vi "CS POLARIS BME DG Client.ProcCases.vi"(0 "i ref in":refnum<vi>, 1 "selector":string, 2 "Data":T1, 3 "call cluster":T2={"Object"="", "Selector"="", "CallType"=enum."synchronous", "Async Object"="", "Async Selector"="", "Data Descriptor"="", "Data"=[], "Error #"=0, "Expire"=0}, 5 "error in (no error)":errorcluster) -> (14 "i ref out":refnum<vi>, 17 "answer cluster":T2={"Object"="", "Selector"="", "CallType"=enum."synchronous", "Async Object"="", "Async Selector"="", "Data Descriptor"="", "Data"=[], "Error #"=0, "Expire"=0}, 19 "error out":errorcluster)   [LabVIEW 2009, in "CS POLARIS BME DG Client.lvlib"]
doc: "This method is called by a process from within the default case in the event loop. The methods of a class that are linked to events will be called from THIS method. Add your code here."
uses:
  CS POLARIS BME DG Client.lvlib
  CSCore/CSSystem/CoreDefs/CoreDefs.call_type.ctl
  CSCore/BaseProcess/BaseProcess.descriptor string definition.ctl
  CSCore/CSSystem/CoreDefs/CoreDefs.rawDataType.ctl
  CSCore/BaseProcess/BaseProcess.lvlib
  CSCore/CAEObj/CAEObj.lvlib
  lib.lib/UtilityLib/UtilityLib.lvlib
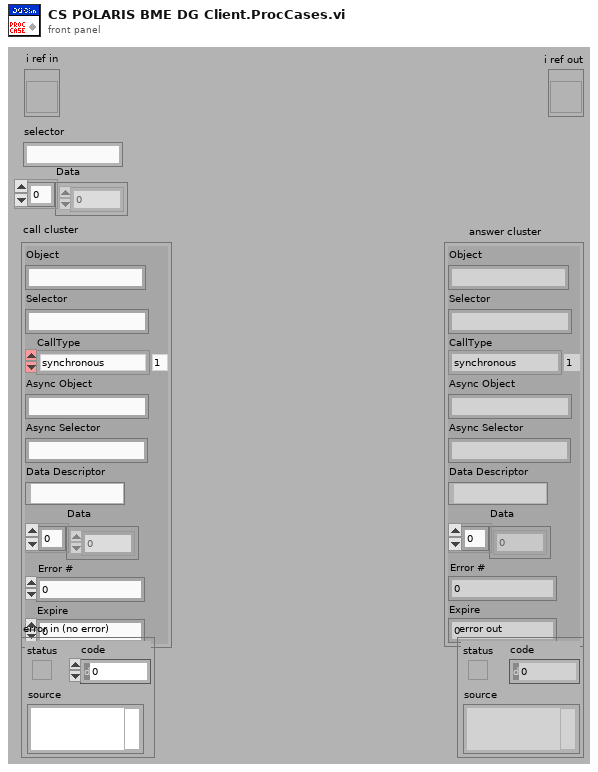
[diagram p1: front panel]
types:
  T1 = typedef "CoreDefs.rawDataType.ctl" = i8[]
  T2 = typedef "CoreDefs.call_type.ctl" = cluster{"Object":string, "Selector":string, "CallType":enum16{"simple", "synchronous", "asynchronous"}, "Async Object":string, "Async Selector":string, "Data Descriptor":T3, "Data":T1, "Error #":i32, "Expire":u32}
  T3 = typedef "BaseProcess.lvlib/BaseProcess.descriptor string definition.ctl" = string
  T4 = typedef "CS POLARIS BME DG Client.lvlib/CS POLARIS BME DG Client.i attribute.ctl" = cluster{"Delay Formula Ref":refnum<vi>, "Active Ref":refnum<vi>, "OutputModulo Ref":refnum<vi>, "Rep Rate Ref":refnum<vi>, "Next Shot Ref":refnum<vi>, "Error Ref":refnum<vi>, "Switch Ref":refnum<vi>, "New Delay Formula Ref":refnum<vi>, "New OutputModulo Ref ":refnum<vi>, "Channel":string, "CS DG Obj":string, "Stop Ref":refnum<vi>, "Max delay change":dbl, "Enabled fields":u8, "LockInfo Ref":refnum<vi>, "Next Common Shot Ref":refnum<vi>, "cur. abs del Ref":refnum<vi>, "new abs del Ref 2":refnum<vi>}
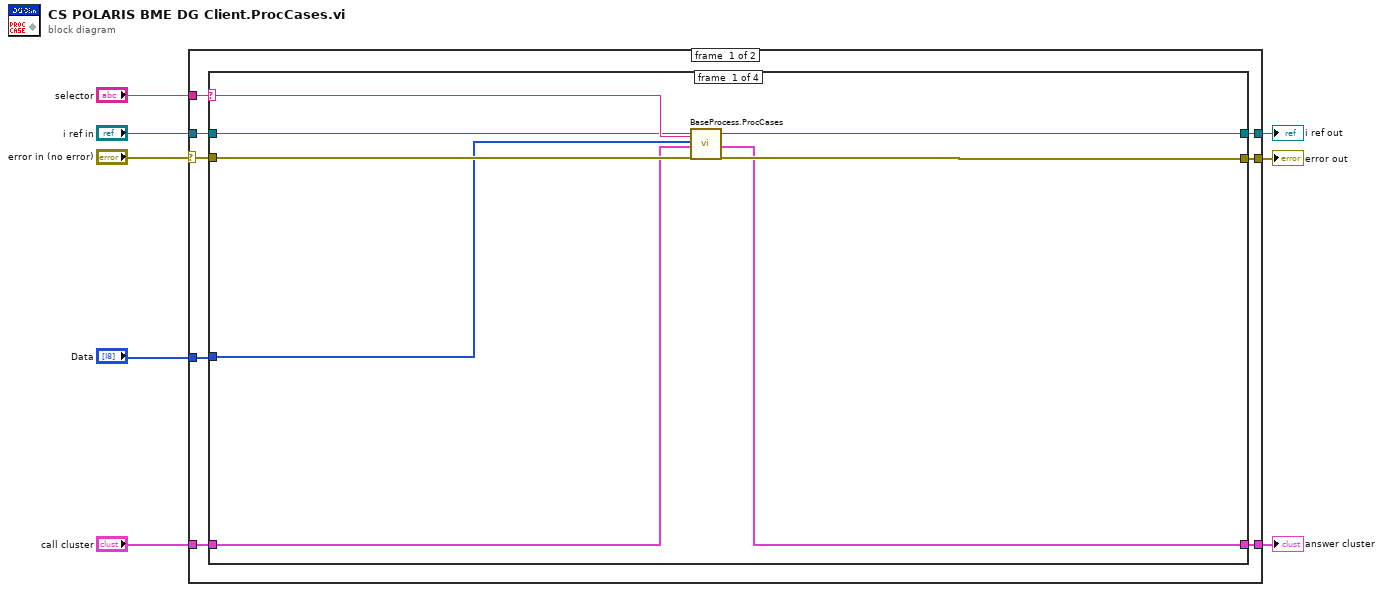
[diagram p0: block diagram]
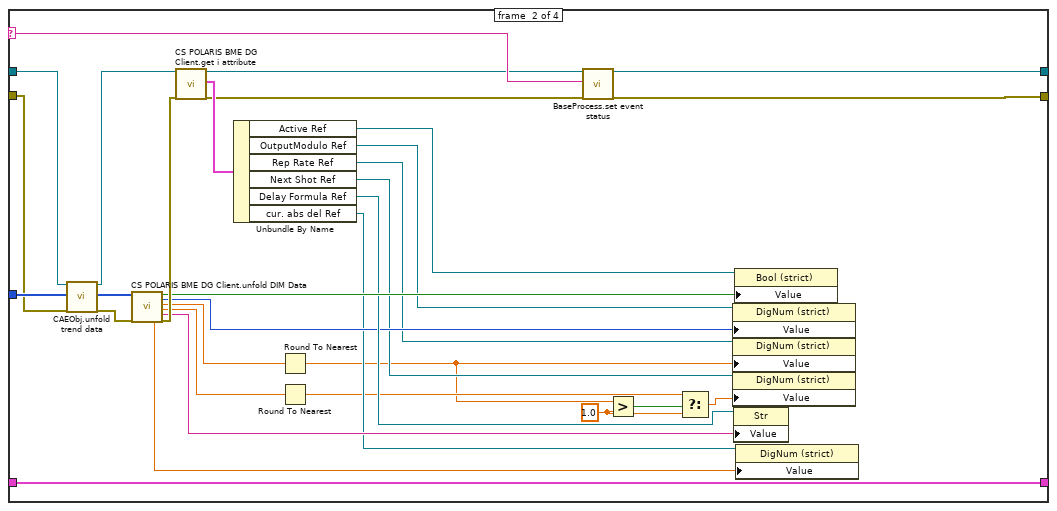
[diagram p2: hidden frame]
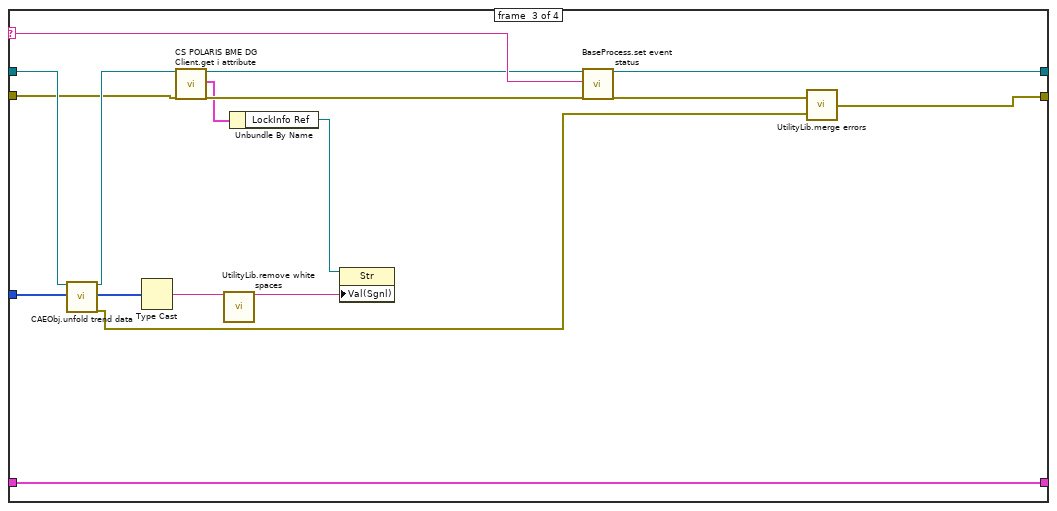
[diagram p3: hidden frame]
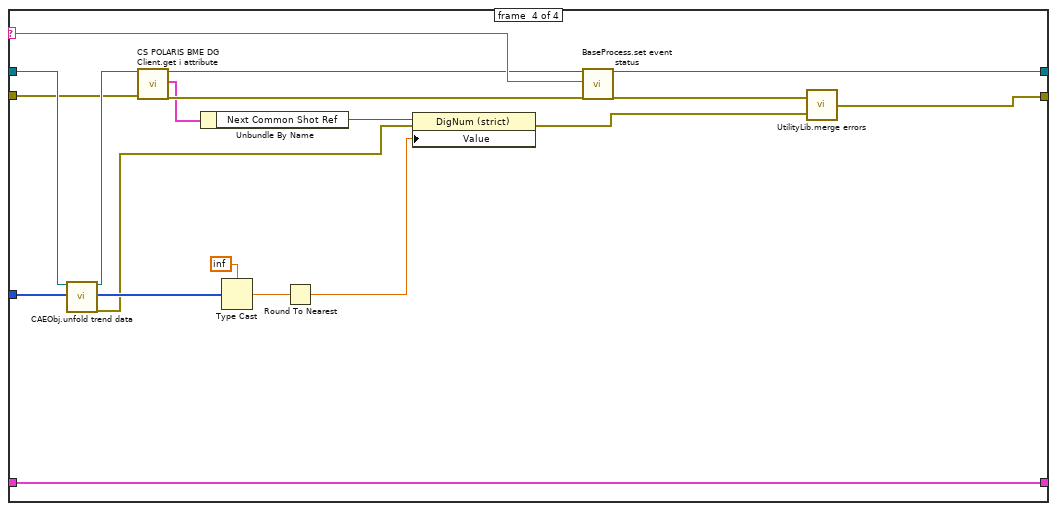
[diagram p4: hidden frame]
diagram:
  n1 = case shown="No Error" "error in (no error)" {
    selector: "error in (no error)" -> [w9 w92]
    tunnel: "selector" -> [w16 _]
    tunnel: [w15 w93] -> w7
    tunnel: "Data" -> [w14 _]
    tunnel: "call cluster" -> [w13 w93]
    tunnel: "i ref in" -> [w12 w94]
    tunnel: [w11 w94] -> w3
    tunnel: [w10 w92] -> w2
    frame #0 {
      n2 = case shown="\"Chnldata\"" w16 {
        selector: w16 -> [w18 w54 w72 w91]
        tunnel: w14 -> [w19 w36 w60 w80]
        tunnel: w12 -> [w17 w35 w67 w86]
        tunnel: [w24 w53 w71 w90] -> w11
        tunnel: w13 -> [w20 w37 w68 w87]
        tunnel: [w21 w37 w68 w87] -> w15
        tunnel: w9 -> [w23 w32 w61 w81]
        tunnel: [w22 w55 w62 w82] -> w10
        frame #0 {
          n3 = call "BaseProcess.ProcCases.vi"("i ref in"=w17, "selector"=w18, "Data"=w19, "call cluster"=w20, "error in (no error)"=w23) -> ("i ref out"=w24:refnum<vi>, "answer cluster"=w21:T2, "error out"=w22:errorcluster)  [unwired: 12 in]
        }
        frame #1 {
          w28 = 1.0 ("f")
          n4 = call "CAEObj.unfold trend data.vi"("i ref in"=w35, "raw trend data"=w36, "error in (no error)"=w32) -> ("i ref out"=w34:refnum<vi>, "data"=w33:i8[], "error out"=w31:errorcluster)  [unwired: 8 in, 6 out]
          n5 = call "CS POLARIS BME DG Client.unfold DIM Data.vi"("Data"=w33, "error in (no error)"=w31) -> ("CurAbsDelay"=w39:dbl, "On"=w48:bool, "output modulo"=w46:i32, "RepRate"=w43:dbl, "NextShot"=w41:dbl, "DelayFormula"=w49:string, "error out"=w51:errorcluster)  [unwired: 11 in]
          n6 = call "CS POLARIS BME DG Client.get i attribute.vi"("i ref in"=w34, "error in (no error)"=w51) -> ("i ref out"=w52:refnum<vi>, "i attribute"=w50:T4, "error out"=w25:errorcluster)  [unwired: 15 in]
          n7 = Unbundle By Name(w50) -> ("Active Ref"=w38:refnum<vi>, "OutputModulo Ref"=w45:refnum<vi>, "Rep Rate Ref"=w44:refnum<vi>, "Next Shot Ref"=w42:refnum<vi>, "Delay Formula Ref"=w47:refnum<vi>, "cur. abs del Ref"=w40:refnum<vi>)
          n8 = Round To Nearest(number=w43) -> (nearest integer value=w26:dbl)
          n9 = Round To Nearest(number=w41) -> (nearest integer value=w29:dbl)
          n10 = call "BaseProcess.set event status.vi"("i ref in"=w52, "EventStatus"=w54, "error in (no error)"=w25) -> ("i ref out"=w53:refnum<vi>, "error out"=w55:errorcluster)  [unwired: 14 in, 1 out]
          n11 = Greater?(x=w26, y=w28) -> (0:w27:bool)
          n12 = Select(t=w29, s=w27, f=w28) -> (s? t:f=w30:dbl)
          n13 = property class="DigNum (strict)"(reference=w45, "Value"=w46) -> ()  [unwired: 1 in, 2 out]
          n14 = property class="DigNum (strict)"(reference=w44, "Value"=w26) -> ()  [unwired: 1 in, 2 out]
          n15 = property class="DigNum (strict)"(reference=w42, "Value"=w30) -> ()  [unwired: 1 in, 2 out]
          n16 = property class="Str"(reference=w47, "Value"=w49) -> ()  [unwired: 1 in, 2 out]
          n17 = property class="Bool (strict)"(reference=w38, "Value"=w48) -> ()  [unwired: 1 in, 2 out]
          n18 = property class="DigNum (strict)"(reference=w40, "Value"=w39) -> ()  [unwired: 1 in, 2 out]
        }
        frame #2 {
          n19 = call "CAEObj.unfold trend data.vi"("i ref in"=w67, "raw trend data"=w60) -> ("i ref out"=w66:refnum<vi>, "data"=w58:i8[], "error out"=w59:errorcluster)  [unwired: 9 in, 6 out]
          n20 = Type Cast(x=w58) -> (*(type *) &x=w57:string)  [unwired: 1 in]
          n21 = call "CS POLARIS BME DG Client.get i attribute.vi"("i ref in"=w66, "error in (no error)"=w61) -> ("i ref out"=w70:refnum<vi>, "i attribute"=w65:T4, "error out"=w69:errorcluster)  [unwired: 15 in]
          n22 = call "UtilityLib.remove white spaces.vi"("string with blanks"=w57) -> ("string without white spaces"=w56:string)  [unwired: 14 in, 4 out]
          n23 = Unbundle By Name(w65) -> ("LockInfo Ref"=w64:refnum<vi>)
          n24 = property class="Str"(reference=w64, "Val(Sgnl)"=w56) -> ()  [unwired: 1 in, 2 out]
          n25 = call "BaseProcess.set event status.vi"("i ref in"=w70, "EventStatus"=w72, "error in (no error)"=w69) -> ("i ref out"=w71:refnum<vi>, "error out"=w63:errorcluster)  [unwired: 14 in, 1 out]
          n26 = call "UtilityLib.merge errors.vi"("error2 (no error)"=w59, "error1 (no error)"=w63) -> ("error out"=w62:errorcluster)
        }
        frame #3 {
          n27 = call "CAEObj.unfold trend data.vi"("i ref in"=w86, "raw trend data"=w80) -> ("i ref out"=w85:refnum<vi>, "data"=w79:i8[], "error out"=w74:errorcluster)  [unwired: 9 in, 6 out]
          n28 = call "CS POLARIS BME DG Client.get i attribute.vi"("i ref in"=w85, "error in (no error)"=w81) -> ("i ref out"=w89:refnum<vi>, "i attribute"=w84:T4, "error out"=w88:errorcluster)  [unwired: 15 in]
          n29 = Unbundle By Name(w84) -> ("Next Common Shot Ref"=w77:refnum<vi>)
          n30 = Type Cast(type=inf, x=w79) -> (*(type *) &x=w76:dbl)
          n31 = Round To Nearest(number=w76) -> (nearest integer value=w75:dbl)
          n32 = property class="DigNum (strict)"(reference=w77, error in=w74, "Value"=w75) -> (error out=w73:errorcluster)  [unwired: 1 out]
          n33 = call "BaseProcess.set event status.vi"("i ref in"=w89, "EventStatus"=w91, "error in (no error)"=w88) -> ("i ref out"=w90:refnum<vi>, "error out"=w83:errorcluster)  [unwired: 14 in, 1 out]
          n34 = call "UtilityLib.merge errors.vi"("error2 (no error)"=w73, "error1 (no error)"=w83) -> ("error out"=w82:errorcluster)
        }
      }
    }
    frame #1 {
    }
  }
  "answer cluster" <- w7
  "i ref out" <- w3
  "error out" <- w2
